vi "Recall Memory Location Values.vi"(8 "error in (no error)":errorcluster, 10 "Preset":i32(ring) items=["Preset1", "Preset2", "Preset3"], 11 "VISA resource name":refnum<visa-resource-name>) -> (0 "error out":errorcluster, 3 "VISA resource name out":refnum<visa-resource-name>)   [LabVIEW 2021, in "BK Precision 169XB.lvlib"]
doc: "Returns the actual voltage level and actual current level for a desired channel."
uses:
  BK Precision 169XB.lvlib
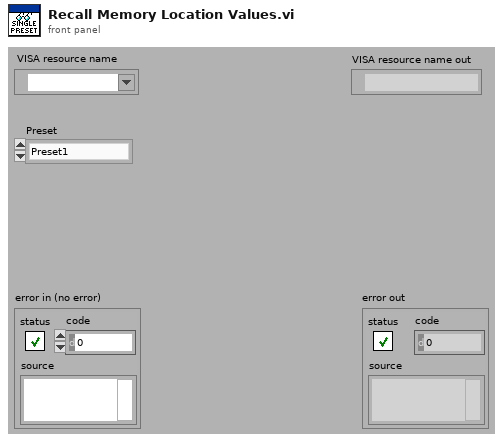
[diagram p1: front panel]
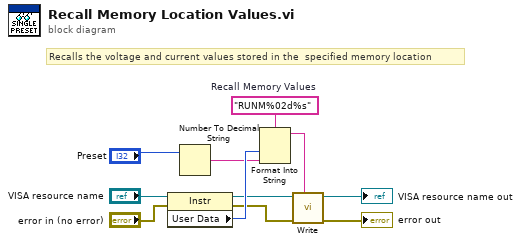
[diagram p0: block diagram]
diagram:
  w8 = "RUNM%02d%s"  # Recall Memory Values
  # "Recalls the voltage and current values stored in the  specified memory location"
  n1 = property class="Instr"(reference="VISA resource name", error in="error in (no error)") -> (reference out=w4:refnum<visa-resource-name>, error out=w3:errorcluster, "User Data"=w7:u32)
  n2 = Number To Decimal String(number="Preset") -> (decimal integer string=w6:string)  [unwired: 1 in]
  n3 = Format Into String(format string=w8, w7, w6) -> (resulting string=w1:string)  [unwired: 2 in, 1 out]
  n4 = call "Write.vi"("Input String"=w1, "error in (no error)"=w3, "VISA resource name"=w4) -> ("error out"=→"error out":errorcluster, "VISA resource name out"=→"VISA resource name out":refnum<visa-resource-name>)  [unwired: 6 in, 1 out]
